vi "GetPowerSpectrum.vi"(6 "calc cache":variant, 11 "Waveform":waveform(sgl)) -> (1 "spectrum info":T1={"channel name"="", "description"="", "x-axis units"=0, "spectral info"={"spectrum type"=enum."Power [Magnitude^2]", "linear/dB"=enum."linear", "window"=0, "window size"=0, "FFT size"=0}, "engineering units"=0, "custom label"="", "dB reference [EU]"=0.0, "peak units"=enum."rms", "weighting filter"=0, "spectral density?"=FALSE, "unit label"="", "spectrum skewed?"=FALSE, "complimentary spectrum units"=enum."none"} {"x-axis units" items=["Time (s)"=0, "Frequency-CB (Hz)"=1, "Frequency-CPB (Hz)"=1248, "Frequency-Arbitrary (Hz)"=2357, "Quefrency (s)"=2, "Revolutions (rev)"=3, "Order"=4, "Speed (RPM)"=11, "Speed (rad/s)"=21, "Index"=65535]; "weighting filter" items=["Linear", "A-weighting", "B-weighting", "C-weighting", "ITU-R 468-4", "Dolby", "CCITT", "C-message", "Wb", "Wc", "Wd", "We", "Wf", "Wh", "Wj", "Wk", "Wm", "AES17 20 kHz lowpass", "AES17 40 kHz lowpass", "AES17 20 kHz highpass", "AES17 40 kHz highpass"]; "dB reference [EU]" format="%.2f"; "engineering units" items=["custom..."=0, "V"=1, "A"=21, "C"=30, "pC"=31, "s"=32, "-"=29, "Pa"=2, "N"=20, "g"=3, "m/s^2"=4, "m/s"=5, "m"=6, "mm/s"=12, "mm"=13, "micron/s"=14, "micron"=15, "in/s^2"=7, "in/s"=8, "in"=9, "mil/s"=10, "mil"=11, "rad/s^2"=16, "rad/s"=17, "rad"=18, "deg/s^2"=26, "deg/s"=27, "deg"=28, "RPM"=22, "cycle/s^2"=23, "Hz"=24, "cycle"=25, "strain"=19]; "spectral info"."window" items=["None "=0, "Hanning"=1, "Hamming"=2, "Blackman-Harris"=3, "Exact Blackman"=4, "Blackman"=5, "Flat Top"=6, "4 Term B-Harris "=7, "7 Term B-Harris"=8, "Low Sidelobe"=9, "Force - Exponential"=10, "Gaussian"=62]}, 3 "power spectrum [EU^2 rms]":cluster{"f0":dbl, "df":dbl, "magnitude":sgl[]} {"magnitude" format="%.2p"; "df" format="%.2p"; "f0" format="%.2p"}, 4 "calc cache out":variant)   [LabVIEW 2017, in "AnalysisHelper.lvlib"]
uses:
  <vilib>/addons/InsightCM/Utilities/Analysis/Shared/AnalysisHelper.lvlib
  <vilib>/addons/_NISVFA/_Shared subVIs/Controls/svc_Spectrum Info.ctl
  <vilib>/addons/_NISVFA/_Shared subVIs/Controls/svc_X-Axis Units.ctl
  <vilib>/addons/_NISVFA/_Shared subVIs/Controls/svc_Spectrum Type.ctl
  <vilib>/addons/_NISVFA/_Shared subVIs/Controls/svc_Engineering Units Text Ring.ctl
  <vilib>/addons/_NISVFA/_Shared subVIs/Controls/svc_Weighting Filter Text Ring.ctl
  <vilib>/addons/_NISVFA/_Shared subVIs/Controls/svc_Complimentary Spectrum Units.ctl
  <vilib>/addons/InsightCM/Utilities/Analysis/Vibration/VibrationAnalysisFunctions.lvlib
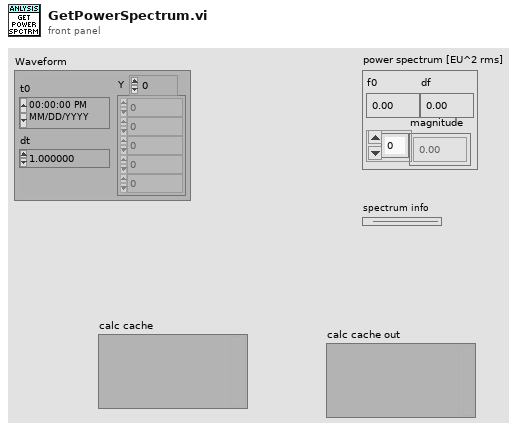
[diagram p1: front panel]
types:
  T1 = typedef "svc_Spectrum Info.ctl" = cluster{"channel name":string, "description":string, "x-axis units":T2, "spectral info":cluster{"spectrum type":T3, "linear/dB":enum16{"linear", "dB"}, "window":u16, "window size":i32, "FFT size":i32}, "engineering units":T4, "custom label":string, "dB reference [EU]":dbl, "peak units":enum16{"rms", "peak", "peak-peak"}, "weighting filter":T5, "spectral density?":bool, "unit label":string, "spectrum skewed?":bool, "complimentary spectrum units":T6}
  T2 = typedef "svc_X-Axis Units.ctl" = u16
  T3 = typedef "svc_Spectrum Type.ctl" = enum16{"FFT Spectrum [complex]", "Amplitude [Magnitude]", "Power [Magnitude^2]", "Cross Spectrum [complex]", "Frequency Response [Complex]"}
  T4 = typedef "svc_Engineering Units Text Ring.ctl" = u16
  T5 = typedef "svc_Weighting Filter Text Ring.ctl" = u16
  T6 = typedef "svc_Complimentary Spectrum Units.ctl" = enum16{"none", "radians", "degrees", "cycles", "imaginary"}
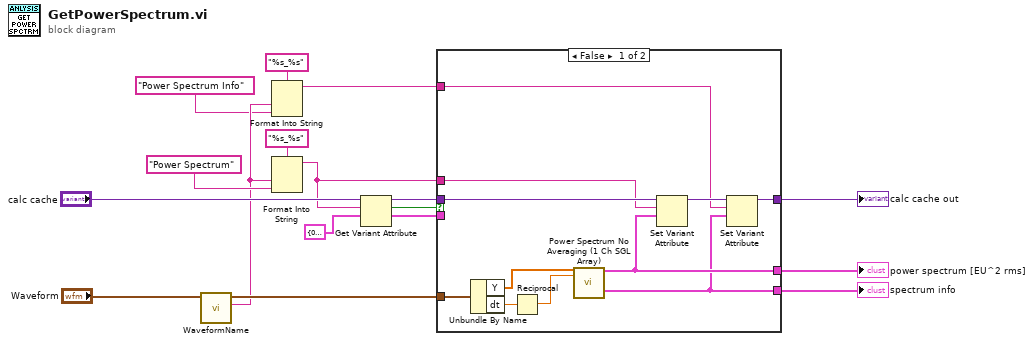
[diagram p0: block diagram]
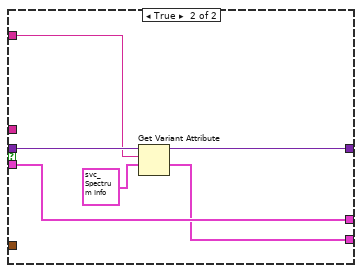
[diagram p2: hidden frame]
diagram:
  n1 = call <vilib>:"WaveformName.vi"("signal in"="Waveform") -> ("name"=w3:string, "signal out"=w8:waveform(sgl))  [unwired: 9 in]
  n2 = Format Into String(format string="%s_%s", w3, "Power Spectrum Info" ("name")) -> (resulting string=w4:string)  [unwired: 2 in, 1 out]
  n3 = Format Into String(format string="%s_%s", w3, "Power Spectrum" ("name")) -> (resulting string=w5:string)  [unwired: 2 in, 1 out]
  n4 = Get Variant Attribute(Variant="calc cache", name=w5, default value (empty Variant)=cluster{"f0":dbl, "df":dbl, "magnitude":sgl[]} {"f0"=0.0, "df"=0.0, "magnitude"=[]} ("power spectrum [EU^2 rms]")) -> (duplicate Variant=w11:variant, found=w13:bool, value=w12:cluster{"f0":dbl, "df":dbl, "magnitude":sgl[]})  [unwired: 1 in, 1 out]
  n5 = case shown="False" w13 {
    tunnel: w8 -> [w26 _]
    tunnel: [w22 w34] -> w17
    tunnel: [w19 w31] -> w16
    tunnel: w12 -> [_ w34]
    tunnel: w11 -> [w24 w33]
    tunnel: [w18 w30] -> w10
    tunnel: w5 -> [w23 _]
    tunnel: w4 -> [w20 w29]
    frame False {
      n6 = Unbundle By Name(w26) -> ("Y"=w25:sgl[], "dt"=w27:dbl)
      n7 = Reciprocal(x=w27) -> (1/x=w28:dbl)
      n8 = call <vilib>:"Power Spectrum No Averaging (1 Ch SGL Array).vi"("scaled signal [EU]"=w25, "sampling rate [Hz]"=w28) -> ("power spectrum [EU^2 rms]"=w22:cluster{"f0":dbl, "df":dbl, "magnitude":sgl[]}, "spectrum info"=w19:T1)  [unwired: 16 in]
      n9 = Set Variant Attribute(Variant=w24, name=w23, value=w22) -> (Variant out=w21:variant)  [unwired: 1 in, 2 out]
      n10 = Set Variant Attribute(Variant=w21, name=w20, value=w19) -> (Variant out=w18:variant)  [unwired: 1 in, 2 out]
    }
    frame True {
      n11 = Get Variant Attribute(Variant=w33, name=w29, default value (empty Variant)=T1 {"channel name"="", "description"="", "x-axis units"=0, "spectral info"={"spectrum type"=enum."Power [Magnitude^2]", "linear/dB"=enum."linear", "window"=0, "window size"=0, "FFT size"=0}, "engineering units"=1, "custom label"="", "dB reference [EU]"=0.0, "peak units"=enum."rms", "weighting filter"=0, "spectral density?"=FALSE, "unit label"="", "spectrum skewed?"=FALSE, "complimentary spectrum units"=enum."none"} ("spectrum info")) -> (duplicate Variant=w30:variant, value=w31:T1)  [unwired: 1 in, 2 out]
    }
  }
  "power spectrum [EU^2 rms]" <- w17
  "spectrum info" <- w16
  "calc cache out" <- w10
